vi "Mixer Calc.vi"(4 "Mixer Type":u16(ring)=2 items=["LO<RF", "LO>RF", "Automatic"], 6 "Lo Freq":dbl, 11 "IN Freq":dbl) -> (1 "OUT LOW":dbl, 2 "OUT HIGH":dbl)   [LabVIEW 2018]
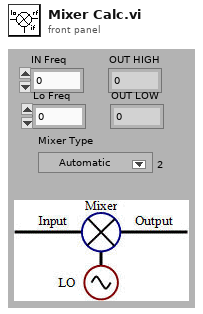
[diagram p1: front panel]
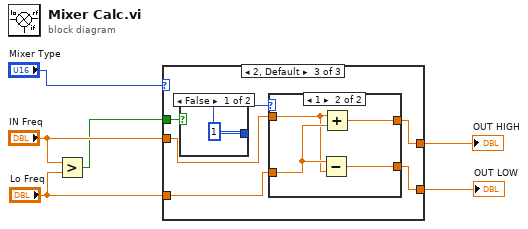
[diagram p0: block diagram]
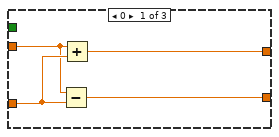
[diagram p2: hidden frame]
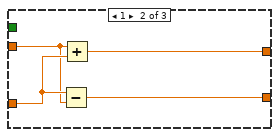
[diagram p3: hidden frame]
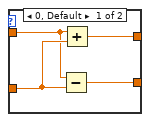
[diagram p4: hidden frame]
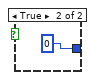
[diagram p5: hidden frame]
diagram:
  n1 = Greater?(x="IN Freq", y="Lo Freq") -> (0:w1:bool)
  n2 = case shown="2, Default" "Mixer Type" {
    tunnel: [w10 w14 w19] -> w6
    tunnel: [w9 w13 w18] -> w5
    tunnel: "IN Freq" -> [w7 w11 w17]
    tunnel: "Lo Freq" -> [w8 w12 w16]
    tunnel: w1 -> [_ _ w15]
    frame 0 {
      n3 = Subtract(x=w7, y=w8) -> (x-y=w9:dbl)
      n4 = Add(x=w7, y=w8) -> (x+y=w10:dbl)
    }
    frame 1 {
      n5 = Subtract(x=w12, y=w11) -> (x-y=w13:dbl)
      n6 = Add(x=w11, y=w12) -> (x+y=w14:dbl)
    }
    frame 2, Default {
      n7 = case shown="False" w15 {
        tunnel: [1 0] -> w20
        frame False {
        }
        frame True {
        }
      }
      n8 = case shown="1" w20 {
        tunnel: [w24 w28] -> w19
        tunnel: [w23 w27] -> w18
        tunnel: w17 -> [w21 w25]
        tunnel: w16 -> [w22 w26]
        frame 0, Default {
          n9 = Subtract(x=w21, y=w22) -> (x-y=w23:dbl)
          n10 = Add(x=w21, y=w22) -> (x+y=w24:dbl)
        }
        frame 1 {
          n11 = Subtract(x=w26, y=w25) -> (x-y=w27:dbl)
          n12 = Add(x=w25, y=w26) -> (x+y=w28:dbl)
        }
      }
    }
  }
  "OUT HIGH" <- w6
  "OUT LOW" <- w5
